vi "dms-main-train-1.vi"() -> ()   [LabVIEW 2015]
uses:
  states-enum.ctl
  <vilib>/platform/TimedLoop/XDataNode/XDataNode.xnode
  <vilib>/Platform/TimedLoop/XDataNode/nitl_modes.ctl
  <vilib>/Platform/TimedLoop/XDataNode/XDNodeRunTimeDep.lvlib
  <vilib>/Platform/TimedLoop/XDataNode/wakeup.ctl
  <vilib>/Platform/TimedLoop/XDataNode/timing_clust.ctl
  Device/Methods/Speaker-Play.vi
  Rack/Methods/Rack-Refresh.vi
  Device/Methods/Lickometer-Read.vi
  Device/Methods/Valve-Init.vi
  Device/Methods/Juicer-Init.vi
  Device/Methods/Speaker-Init.vi
  Rack/Methods/Rack-Start.vi
  Rack/Methods/Rack-Config.vi
  Device/Methods/Lickometer-Init.vi
  Rack/Methods/Rack-Init.vi
  Device/Methods/Valve-Pulse.vi
  <vilib>/Utility/file.llb/Read Delimited Spreadsheet (I64).vi
  Device/Methods/Lickometer-Stop.vi
  Rack/Methods/Rack-Stop.vi
  Rack/Typedefs/OutputRequest.ctl
  Rack/Typedefs/OutputRequest refnum.ctl
  Rack/Methods/Port drivers/DigitalInput-DataCluster.ctl
  Rack/Typedefs/InputData cluster.ctl
  Device/Typedefs/Lickometer.ctl
  Device/Typedefs/Speaker.ctl
  Device/Typedefs/Juicer.ctl
  Device/Typedefs/Valve.ctl
panel:
  out "InputData 3":T1
  out "InputData 2":T1
  in  "stop":bool
  out "Acc":dbl
  out "Time":dbl format="%#.0f"
  out "Trials":string
  out "Reward Dispensed (uL)":string
  out "Licks":string
  out "CR":string
  out "Miss":string
  out "FA":string
  out "Hits":string
  out "Current State":string
  out "Time Elapsed":dbl format="%<%H:%M:%S>t"
  in  "Tab Control":enum32{"Required", "Optional", "Devices"}(tab)
  in  "Tone Pairs":u16(ring) items=["1: 3000 Hz, 12000 Hz", "2: 5800 Hz, 5000 Hz", "3: 5000 Hz, 10000 Hz", "4: 8000 Hz, 15000 Hz"]
  in  "Max Time (s)":dbl=3600.0
  in  "Number of trials":string(combo)="500"
  in  "Max number of \nconsecutive trials":string(combo)="3"
  in  "Animal Name":string="Mouse"
  in  "Reward Vol. (uL)":dbl=5.0
  in  "Sequence Directory":path=path "C:/Users/SiapasLab/Desktop/git/wheatley"
  in  "Assay Description":string="Auditory delayed match to sample"
  in  "Recording Location":string="BI Room 146"
  in  "Trial delay (ms)":dbl=1500.0
  in  "Punish Time (s)":dbl
  in  "Trial window (ms)":dbl=1000.0
  in  "ITI lower (s)":dbl=10.0
  in  "ITI upper (s)":dbl=10.0
  in  "Min Licks":i32=1 min=1
  in  "Data Saving Directory":path=path "\\\\CA1-17\\ld8007/anesthesia/data"
  in  "Lickometer":T3={"Settings"={"Min lick duration"=1, "Port name"="bnc_panel.p0.3", "Port index"=0}, "Lick"=FALSE, "Debouncing"={"Semaphore"=refnum, "Lick start"=0}, "OutputRequest event ref"=refnum, "InputData reference"=refnum, "Active hi?"=FALSE}
  out "InputData":T1
  in  "Speaker":T6={"Settings"={"Portname"="BNC_Panel.ao0", "Index"=0, "Timestamp portname"="BNC_Panel.P0.0"}, "OutputRequest event ref"=refnum, "InputData reference"=refnum}
  in  "Juicer":T7={"Mode"=enum."Juice/reward", "Settings"={"Bleed #1 port index"=1, "Bleed #1 port name"="juicer.bleed1", "Bleed #2 port name"="juicer.bleed2", "Bleed #2 port index"=2, "Flush port name"="juicer.flush", "Flush port index"=3, "Purge port name"="juicer.purge", "Purge port index"=0, "Timestamp port name"="dsub_panel.p9.7"}, "OutputRequest event ref"=refnum, "InputData reference"=refnum}
  in  "Valve":T8={"Settings"={"Timestamp port name"="BNC_panel.P0.0", "Port name"="BNC_panel.P0.1", "Port index"=4}, "OutputRequest event ref"=refnum, "InputData reference"=refnum, "Default length (ms)"=100}
  # "Auditory delayed match to sample task (DMS)"
  # "(must be on same NI card)"
  # "(must be on same NI card)"
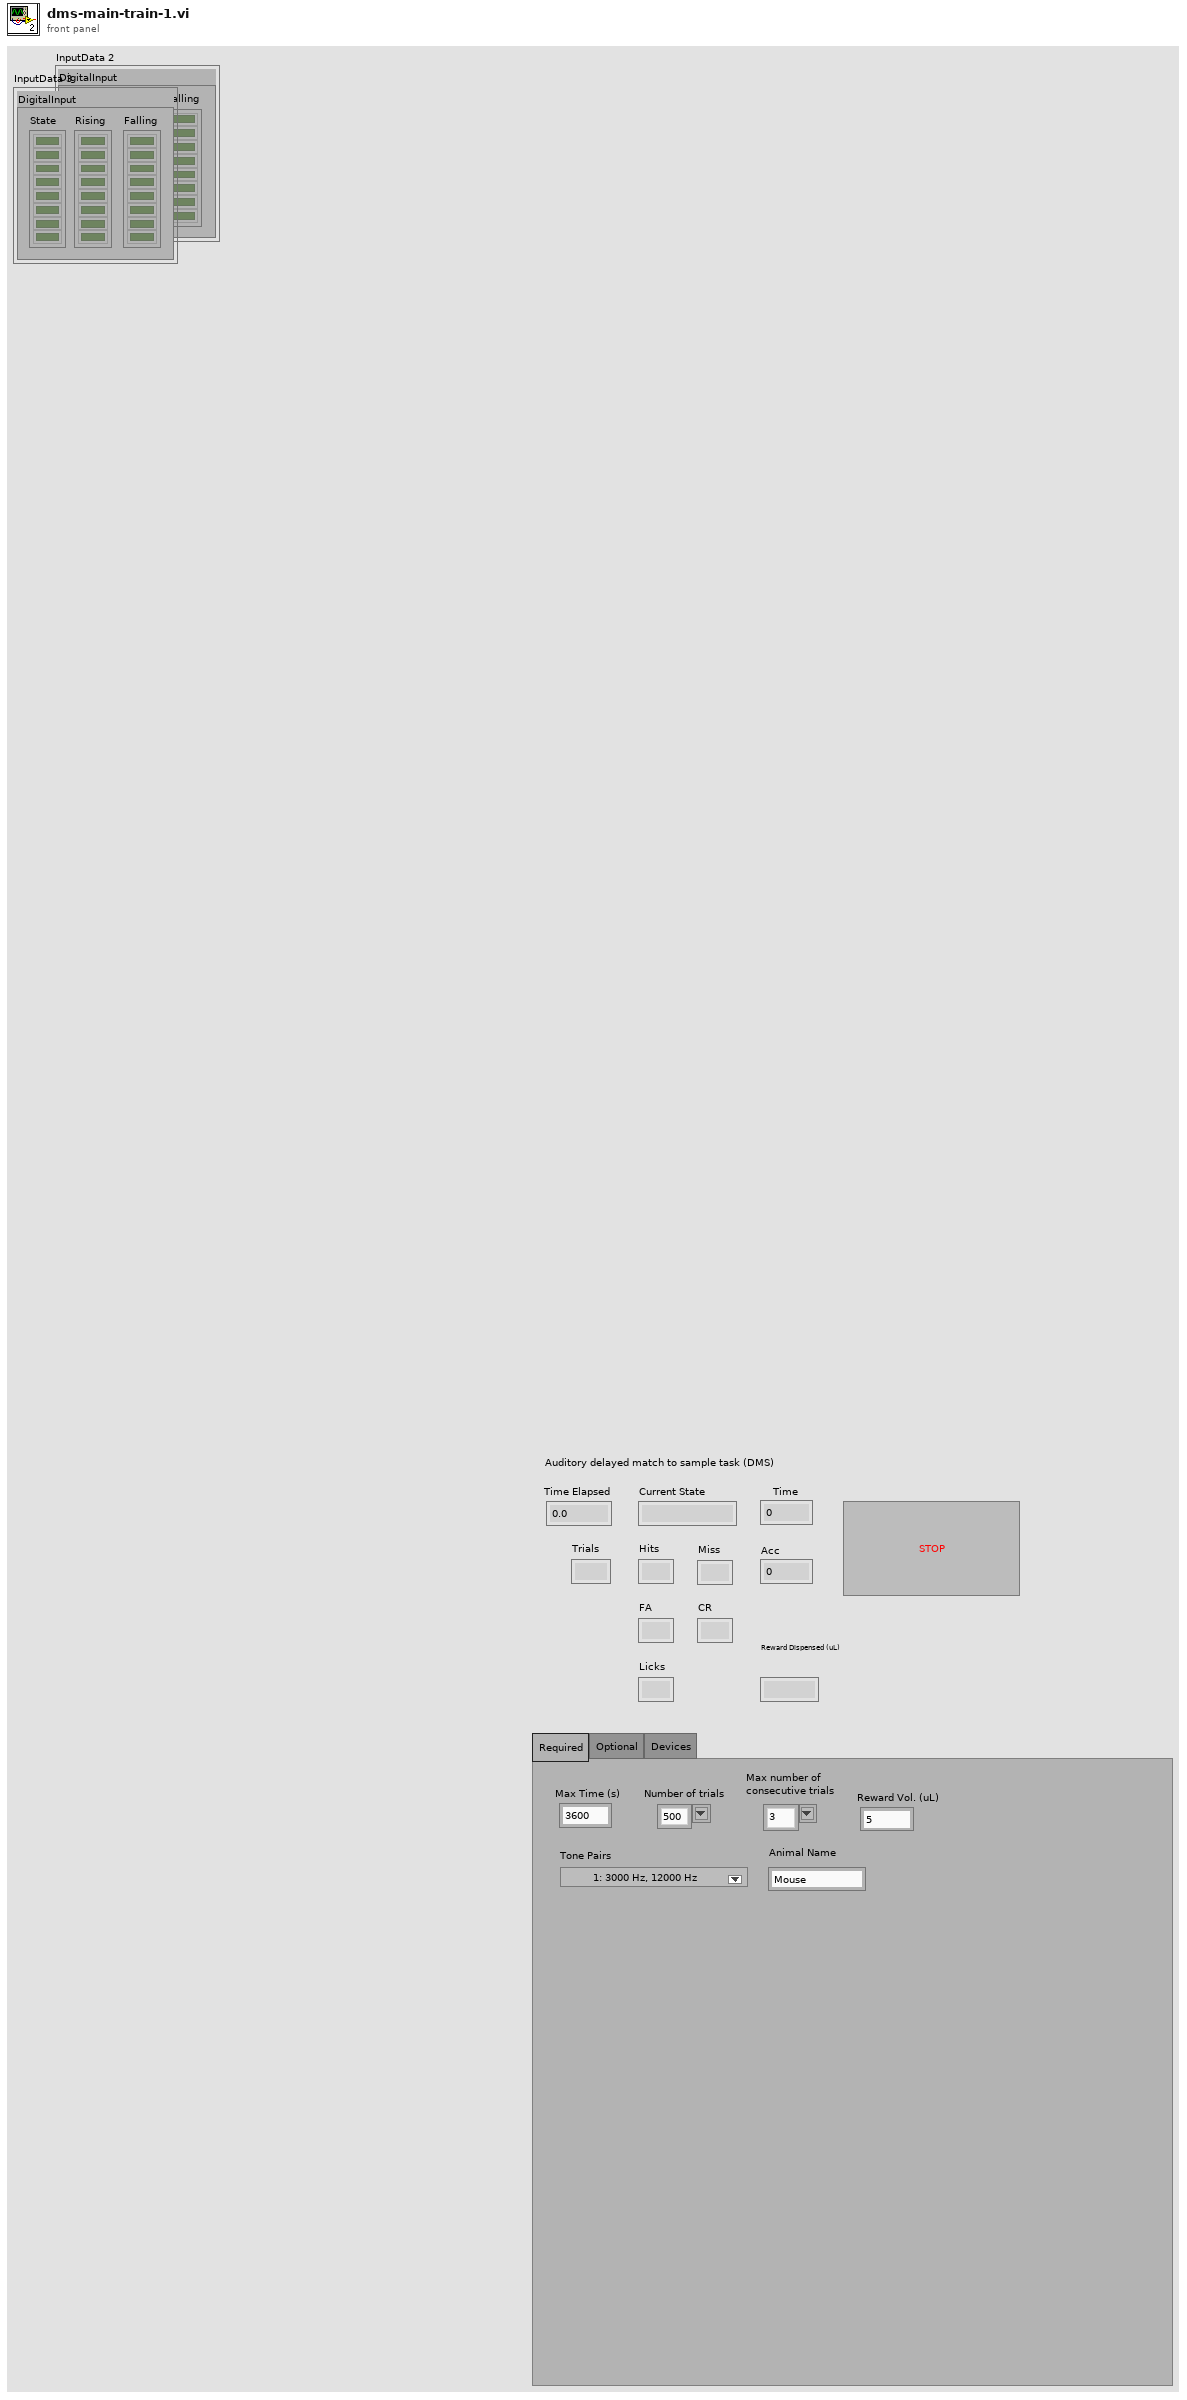
[diagram p1: front panel]
types:
  T1 = typedef "InputData cluster.ctl" = cluster{"DigitalInput":T2}
  T2 = typedef "DigitalInput-DataCluster.ctl" = cluster{"Falling":bool[], "Rising":bool[], "State":bool[]}
  T3 = typedef "Lickometer.ctl" = cluster{"Settings":cluster{"Min lick duration":u32, "Port name":string, "Port index":i32}, "Lick":bool, "Debouncing":cluster{"Semaphore":T4, "Lick start":u32}, "OutputRequest event ref":T5, "InputData reference":refnum<vi>, "Active hi?":bool}
  T4 = typedef "Semaphore RefNum" = refnum<k1>
  T5 = typedef "OutputRequest refnum.ctl" = refnum<user-event>
  T6 = typedef "Speaker.ctl" = cluster{"Settings":cluster{"Portname":string, "Index":i32, "Timestamp portname":string}, "OutputRequest event ref":T5, "InputData reference":refnum<vi>}
  T7 = typedef "Juicer.ctl" = cluster{"Mode":enum16{"Off", "Juice/reward", "Water flush", "Air purge"}, "Settings":cluster{"Bleed #1 port index":i32, "Bleed #1 port name":string, "Bleed #2 port name":string, "Bleed #2 port index":i32, "Flush port name":string, "Flush port index":i32, "Purge port name":string, "Purge port index":i32, "Timestamp port name":string}, "OutputRequest event ref":T5, "InputData reference":refnum<vi>}
  T8 = typedef "Valve.ctl" = cluster{"Settings":cluster{"Timestamp port name":string, "Port name":string, "Port index":i32}, "OutputRequest event ref":T5, "InputData reference":refnum<vi>, "Default length (ms)":i32}
  T9 = typedef "states-enum.ctl" = enum16{"ITI", "Trial", "Stop"}
  T10 = typedef "Rack driver configuration cluster.ctl" = cluster{"DigitalInput":T11, "DigitalOutput":T12, "FileOutput":T13, "AnalogOutput":T14, "DataSocketOutput":T15}
  T11 = typedef "DigitalInput-Configuration.ctl" = cluster{"Lines":tag[], "Refresh period (ms)":u32}
  T12 = typedef "DigitalOutput-Configuration.ctl" = cluster{"Output Lines":tag[], "DO timestamp lines":tag[], "Timestamp lines":tag[]}
  T13 = typedef "FileOutput-Configuration.ctl" = cluster{"Logfile path":path}
  T14 = typedef "AnalogOutput-Configuration.ctl" = cluster{"Output Lines":tag[], "AO timestamp lines":tag[]}
  T15 = typedef "DataSocketOutput-Configuration.ctl" = cluster{"DataSocket URL":string}
  T16 = cluster{"ITI upper (s)":dbl, "ITI lower (s)":dbl, "Punish Time (s)":dbl, "Trial window (ms)":dbl, "Trial delay (ms)":dbl, "Max Time (s)":dbl, "Min Licks":i32, "Reward Vol. (uL)":dbl, "Tone 1":i32, "Tone 2":i32}
  T17 = cluster{"appended path":path, "relative seconds":dbl, "Current Trial Index":i32, "Accuracy":dbl, "Hits":i32, "Miss":i32, "False Alarm":i32, "Correct Rejection":i32, "Licks":i32, "Reward Dispensed":dbl, "Punish ITI":bool, "Next Trial":i32}
  T18 = typedef "XDNodeRunTimeDep.lvlib/timing_clust.ctl" = cluster{"Expected End [f-1]":u64, "Actual End [f-1]":u64, "Finished Late? [f-1]":bool, "Expected End [i-1]":u64, "Actual End [i-1]":u64, "Finished Late? [i-1]":bool, "Expected Start [i]":u64, "Actual Start [i]":u64, "Expected Start [f]":u64, "Actual Start [f]":u64, "Source Name":string, "Structure Name":string, "Period":i64, "Deadline":i64, "Offset":i64, "Start":i64, "Priority":i32, "Timeout":i32, "Mode":T19, "Wakeup Reason":T20, "Error":errorcluster, "Source Type":string, "Secondary Source Type":string, "Global End Time":u64, "Global Start Time":u64, "Frame Duration":u64, "Iteration Duration":u64, "Assigned CPU":i32, "I/O Scan Engine Mode":u32}
  T19 = typedef "XDNodeRunTimeDep.lvlib/nitl_modes.ctl" = enum32{"No Change", "Process missed periods, maintain original phase", "Discard missed periods, maintain original phase", "Process missed periods, ignore original phase", "Discard missed periods, ignore original phase"}
  T20 = typedef "XDNodeRunTimeDep.lvlib/wakeup.ctl" = enum32{"Normal", "Aborted", "Asynchronous wakeup", "Timing source error", "Timed loop error", "Timeout"}
  T21 = cluster{"Trial Hit":bool, "Trial Miss":bool, "Trial FA":bool, "Trial CR":bool, "Skip Receiving":bool}
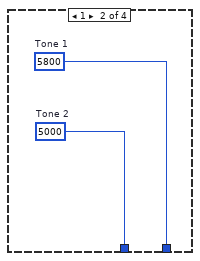
[diagram p2: hidden frame]
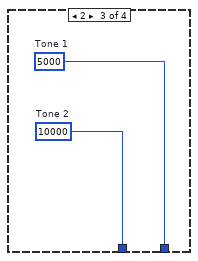
[diagram p3: hidden frame]
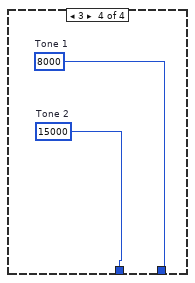
[diagram p4: hidden frame]
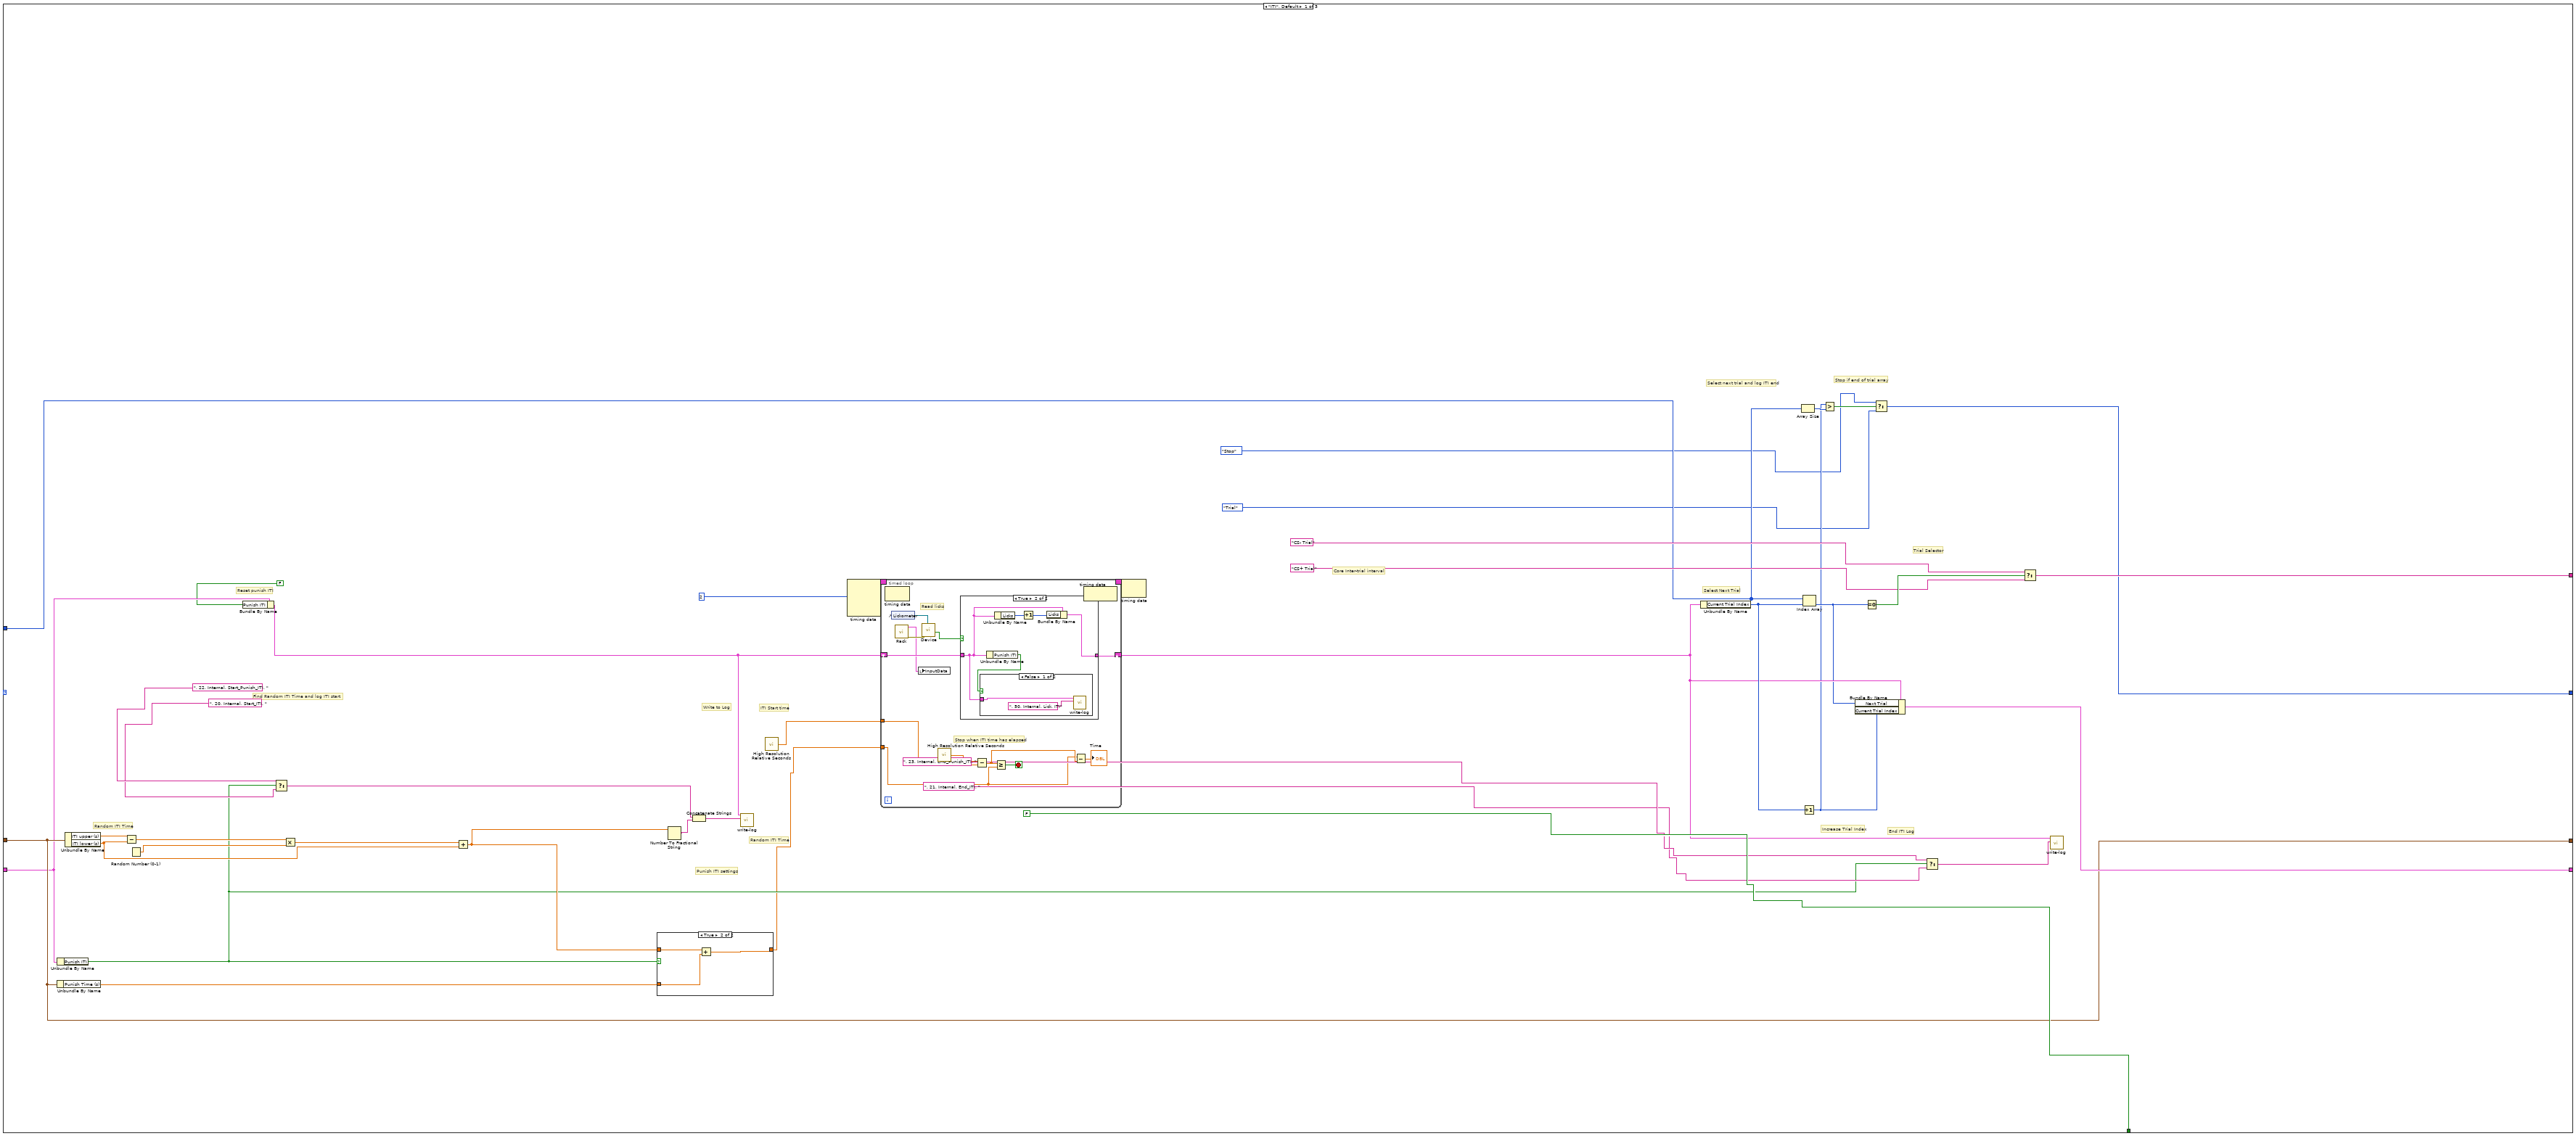
[diagram p6: hidden frame]
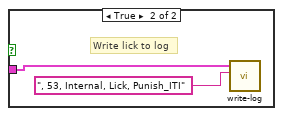
[diagram p8: hidden frame]
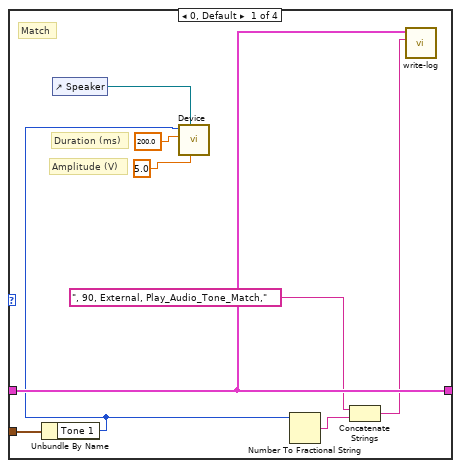
[diagram p11: hidden frame]
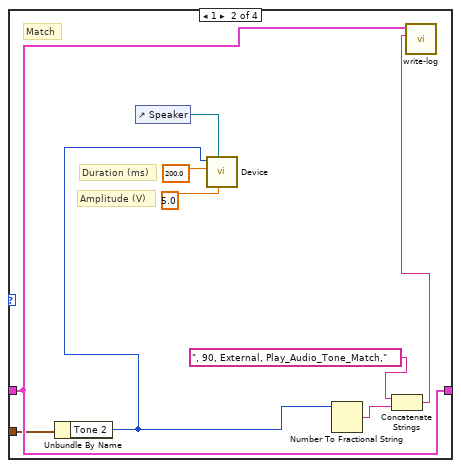
[diagram p12: hidden frame]
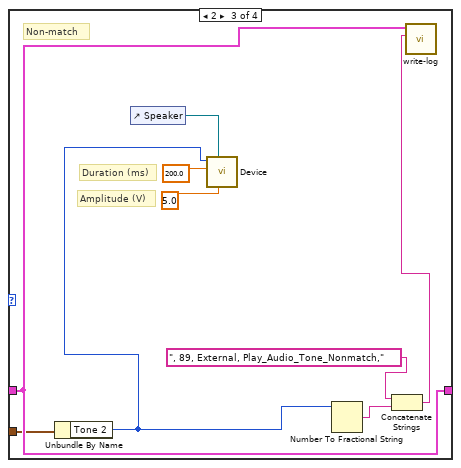
[diagram p13: hidden frame]
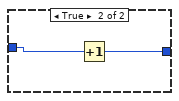
[diagram p14: hidden frame]
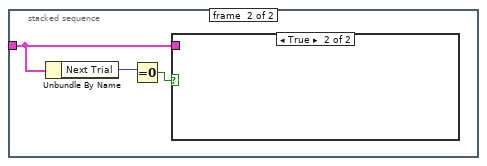
[diagram p16: hidden frame]
diagram:
  w141 = 0  # Next Trial
  w142 = FALSE  # Punish ITI
  w151 = 0.0  # Reward Dispensed
  w152 = 0  # Licks
  w153 = 0  # Correct Rejection
  w154 = 0  # False Alarm
  w157 = 0.0  # Accuracy
  w155 = 0  # Miss
  w156 = 0  # Hits
  w158 = 0  # Current Trial Index
  # "TRAINING"
  # "Create directory"
  # "Lickometer"
  # "Lickometer"
  # "Devices"
  # "Tone Pair Interpretation"
  # "Exit Logging"
  # "Front Panel Logging"
  # "CS+\nDelay lick: Miss\nReception lick: Hit\nNo lick: Miss\n\nCS-\nDelay lick: False alarm\nReception lick: False alarm\nNo lick: Correct reject"
  # "Start time"
  # "Internal Variables"
  # "External variables from Front Panel"
  # "External variable cluster"
  # "Internal variable cluster"
  # "State enum"
  # "Trial shift register"
  # "State machine"
  # "Front Panel Elements"
  # "Write trial sequence to log"
  # "Human readable time"
  # "End of header delimiter"
  # "Start Time"
  # "Environment"
  # "Schedule"
  # "Initialize data logger"
  # "Random sequence selection"
  # "Read in entire .csv"
  # "Load pre-generated sequences"
  n1 = Format Date/Time String(time format string (%c)="%Y-%m-%d-%H-%M-%S") -> (date/time string=w4:string)  [unwired: 2 in]
  n2 = case shown="0, Default" "Tone Pairs" {
    tunnel: [w224 w225 w227 w229] -> w39
    tunnel: [w223 w226 w228 w230] -> w40
    frame 0, Default {
      w224 = 12000  # Tone 2
      w223 = 3000  # Tone 1
    }
    frame 1 {
      w225 = 5000  # Tone 2
      w226 = 5800  # Tone 1
    }
    frame 2 {
      w227 = 10000  # Tone 2
      w228 = 5000  # Tone 1
    }
    frame 3 {
      w229 = 15000  # Tone 2
      w230 = 8000  # Tone 1
    }
  }
  n3 = Build Path(base path="Data Saving Directory", name or relative path=w4) -> (appended path=w2:path)
  n4 = Create Folder(path (use dialog)=w2) -> (created path=w1:path)  [unwired: 2 in, 2 out]
  n5 = control-ref of="InputData"() -> (w13:refnum<vi>)
  n6 = Build Path(base path=w1, name or relative path="data.txt") -> (appended path=w148:path)
  n7 = call-poly "Rack.vi"() -> ("error out"=w7:errorcluster, "OutputRequest\nevent ref"=w8:T5)  [unwired: 10 in]
  n8 = control-ref of="Juicer"() -> (w6:refnum<vi>)
  n9 = Path To String(path="Sequence Directory") -> (string=w96:string)
  n10 = call-poly "Device.vi"("Device reference"=w6, "error in (no error)"=w7, "OutputRequest event ref"=w8, "InputData reference"=w13) -> ("error out"=w10:errorcluster, "OutputRequest (dup)"=w15:T5, "InputData (dup)"=w12:refnum<vi>)  [unwired: 5 in]
  n11 = control-ref of="Valve"() -> (w5:refnum<vi>)
  n12 = Concatenate Strings(w96, "\\sequences\\seq_n_", "Number of trials", "_k_" ("string"), "Max number of \nconsecutive trials", "_m_2.csv" ("string")) -> (w214:string)
  n13 = call-poly "Device.vi"("Device reference"=w5, "error in (no error)"=w10, "OutputRequest event ref"=w15, "InputData reference"=w12) -> ("error out"=w9:errorcluster, "OutputRequest (dup)"=w14:T5, "InputData (dup)"=w11:refnum<vi>)  [unwired: 5 in]
  n14 = String To Path(string=w214) -> (path=w215:path)
  n15 = control-ref of="Speaker"() -> (w16:refnum<vi>)
  n16 = Concatenate Strings("Schedule," ("string"), "Assay Description", "\r\n") -> (w205:string)
  n17 = call-poly "Device.vi"("Device reference"=w16, "error in (no error)"=w9, "OutputRequest event ref"=w14, "InputData reference"=w11) -> ("error out"=w18:errorcluster, "OutputRequest (dup)"=w19:T5, "InputData (dup)"=w17:refnum<vi>)  [unwired: 5 in]
  n18 = Concatenate Strings("Path," ("string"), w96, "\r\n") -> (w99:string)
  n19 = call-poly <vilib>:"Read Delimited Spreadsheet.vi"("file path (dialog if empty)"=w215, "number of rows (all:-1)"=-1, "delimiter (\\t)"="," ("delimiter (\\t)")) -> ("all rows"=w209:i64[][])  [unwired: 7 in, 5 out]
  n20 = Write to Text File(file (use dialog)=w148, text=w205) -> (refnum out=w207:refnum<file>)  [unwired: 2 in, 2 out]
  n21 = control-ref of="Lickometer"() -> (w23:refnum<vi>)
  n22 = call-poly "Device.vi"("Device reference"=w23, "error in (no error)"=w18, "OutputRequest event ref"=w19, "InputData reference"=w17) -> ("error out"=w28:errorcluster, "OutputRequest (dup)"=w25:T5)  [unwired: 5 in, 1 out]
  n23 = Concatenate Strings("Environment," ("string"), "Recording Location", "\r\n") -> (w201:string)
  n24 = Array Size(array=w209) -> (size(s)=w213:i32[])
  n25 = Write to Text File(file (use dialog)=w207, text=w201) -> (refnum out=w101:refnum<file>)  [unwired: 2 in, 2 out]
  n26 = Format Date/Time String() -> (date/time string=w175:string)  [unwired: 3 in]
  n27 = call-poly "Rack.vi"("error in (no error)"=w28) -> ("error out"=w27:errorcluster, "Configuration"=w26:T10)  [unwired: 9 in]
  n28 = Index Array(array=w213, index=0) -> (element=w211:i32)
  n29 = Random Number (0-1)() -> (number: 0 to 1=w220:dbl)
  n30 = Write to Text File(file (use dialog)=w101, text=w99) -> (refnum out=w100:refnum<file>)  [unwired: 2 in, 2 out]
  n31 = Decrement(x=w211) -> (x-1=w210:i32)
  n32 = call-poly "Rack.vi"("error in (no error)"=w27, "OutputRequest event ref"=w25, "Configuration"=w26) -> ("OutputRequest event ref (dup)"=w21:T5)  [unwired: 7 in, 1 out]
  n33 = Multiply(x=w220, y=w210) -> (x*y=w219:dbl)
  n34 = Concatenate Strings("Time," ("string"), w175, "\r\n") -> (w197:string)
  n35 = To Long Integer(number=w219) -> (32bit integer=w208:i32)
  n36 = Write to Text File(file (use dialog)=w100, text=w197) -> (refnum out=w196:refnum<file>)  [unwired: 2 in, 2 out]
  n37 = call <vilib>:"High Resolution Relative Seconds.vi"() -> ("relative seconds"=w160:dbl)
  n38 = Index Array(array=w209, index (row)=w208) -> (element=w150:i64[])  [unwired: 1 in]
  n39 = Bundle("ITI upper (s)"="ITI upper (s)", "ITI lower (s)"="ITI lower (s)", "Punish Time (s)"="Punish Time (s)", "Trial window (ms)"="Trial window (ms)", "Trial delay (ms)"="Trial delay (ms)", "Max Time (s)"="Max Time (s)", "Min Licks"="Min Licks", "Reward Vol. (uL)"="Reward Vol. (uL)", "Tone 1"=w40, "Tone 2"=w39) -> (w135:T16)  [unwired: 1 in]
  n40 = Concatenate Strings("Animal," ("string"), "Animal Name", "\r\n") -> (w193:string)
  n41 = Unbundle By Name(w135) -> ("Max Time (s)"=w134:dbl, "Trial delay (ms)"=w133:dbl, "Trial window (ms)"=w132:dbl, "ITI lower (s)"=w131:dbl, "ITI upper (s)"=w130:dbl, "Punish Time (s)"=w129:dbl, "Min Licks"=w52:i32, "Reward Vol. (uL)"=w44:dbl, "Tone 1"=w32:i32, "Tone 2"=w31:i32)
  n42 = Write to Text File(file (use dialog)=w196, text=w193) -> (refnum out=w185:refnum<file>)  [unwired: 2 in, 2 out]
  n43 = Bundle("appended path"=w148, "relative seconds"=w160, "Current Trial Index"=w158, "Accuracy"=w157, "Hits"=w156, "Miss"=w155, "False Alarm"=w154, "Correct Rejection"=w153, "Licks"=w152, "Reward Dispensed"=w151, "Punish ITI"=w142, "Next Trial"=w141) -> (w159:T17)  [unwired: 1 in]
  n44 = for {
    N -> [w232]
    shift-right: [w236] -> w140
    shift-left: " " -> [w237]
    tunnel: w150 -> [w239] mode=indexing
    i -> [w235]
    n45 = Decrement(x=w232) -> (x-1=w231:i32)
    n46 = Equal?(x=w231, y=w235) -> (x = y?=w234:bool)
    n47 = Number To Decimal String(number=w239) -> (decimal integer string=w238:string)  [unwired: 1 in]
    n48 = case shown="False" w234 {
      tunnel: [", " ("string") "" ("string")] -> w233
      frame False {
      }
      frame True {
      }
    }
    n49 = Concatenate Strings(w237, w238, w233) -> (w236:string)
  }
  n50 = Concatenate Strings("Trials," ("string"), "Number of trials", "\r\n") -> (w189:string)
  n51 = Write to Text File(file (use dialog)=w185, text=w189) -> (refnum out=w184:refnum<file>)  [unwired: 2 in, 2 out]
  n52 = Number To Fractional String(number=w32) -> (F-format string=w33:string)  [unwired: 3 in]
  n53 = Number To Fractional String(number=w44) -> (F-format string=w43:string)  [unwired: 3 in]
  n54 = Number To Fractional String(number=w31) -> (F-format string=w34:string)  [unwired: 3 in]
  n55 = Number To Fractional String(number=w134) -> (F-format string=w128:string)  [unwired: 3 in]
  n56 = Number To Fractional String(number=w129) -> (F-format string=w116:string)  [unwired: 3 in]
  n57 = Number To Fractional String(number=w52) -> (F-format string=w51:string)  [unwired: 3 in]
  n58 = Number To Fractional String(number=w133) -> (F-format string=w125:string)  [unwired: 3 in]
  n59 = Number To Fractional String(number=w132) -> (F-format string=w122:string)  [unwired: 3 in]
  n60 = Number To Fractional String(number=w131) -> (F-format string=w121:string)  [unwired: 3 in]
  n61 = Number To Fractional String(number=w130) -> (F-format string=w119:string)  [unwired: 3 in]
  n62 = Concatenate Strings("Max_Time_s," ("string"), w128, "\r\n") -> (w110:string)
  n63 = Concatenate Strings("Consecutive_Trials," ("string"), "Max number of \nconsecutive trials", "\r\n") -> (w186:string)
  n64 = Concatenate Strings("CS+_Tone," ("string"), w33, "\r\n") -> (w30:string)
  n65 = Concatenate Strings("Min_Licks," ("string"), w51, "\r\n") -> (w48:string)
  n66 = Concatenate Strings("Reward_Volume," ("string"), w43, "\r\n") -> (w42:string)
  n67 = Concatenate Strings("CS-_Tone," ("string"), w34, "\r\n") -> (w29:string)
  n68 = Concatenate Strings("Delay_Window_ms," ("string"), w125, "\r\n") -> (w109:string)
  n69 = Concatenate Strings("ITI_Lower_s," ("string"), w121, "\r\n") -> (w107:string)
  n70 = Concatenate Strings("Reception_Window_ms," ("string"), w122, "\r\n") -> (w108:string)
  n71 = Concatenate Strings("ITI_Upper_s," ("string"), w119, "\r\n") -> (w106:string)
  n72 = Concatenate Strings("Punish_Time_s," ("string"), w116, "\r\n") -> (w105:string)
  n73 = Write to Text File(file (use dialog)=w184, text=w186) -> (refnum out=w104:refnum<file>)  [unwired: 2 in, 2 out]
  n74 = while {
    shift-right: [w275] -> _
    shift-left: states-enum."ITI" -> [w252]
    shift-right: [w251] -> _
    shift-left: w135 -> [w267]
    shift-right: [w266] -> w60
    shift-left: w159 -> [w246]
    tunnel: w150 -> [w269]
    tunnel: w21 -> [w245]
    tunnel: [w245] -> w20
    stop <- w247 stop-if-true
    # "State enum"
    # "Internal variable cluster"
    # "External variable cluster"
    # "Update front panel"
    # "Update front panel"
    # "Wait for current state to finish before ending session"
    n75 = case shown="\"Trial\"" w252 {
      tunnel: [w294 states-enum."ITI" states-enum."Stop"] -> w275
      tunnel: [FALSE FALSE TRUE] -> w271
      tunnel: w269 -> [w299 _ _]
      tunnel: [w303 w403 "Stop"] -> w268
      tunnel: w267 -> [w302 w356 w750]
      tunnel: [w308 w369 w746] -> w266
      tunnel: w246 -> [w293 w372 w746]
      tunnel: [w302 w356 w750] -> w251
      frame "ITI", Default {
        # "Reset punish ITI"
        # "Stop if end of trial array"
        # "Punish ITI settings"
        # "Select next trial and log ITI end"
        # "Trial Selector"
        # "Increase Trial Index"
        # "Select Next Trial"
        # "End ITI Log"
        # "ITI Start time"
        # "Core Inter-trial interval"
        # "Find Random ITI Time and log ITI start"
        # "Random ITI Time"
        # "Write to Log"
        # "Random ITI Time"
        n76 = Unbundle By Name(w302) -> ("Punish Time (s)"=w301:dbl)
        n77 = Unbundle By Name(w293) -> ("Punish ITI"=w284:bool)
        n78 = Unbundle By Name(w302) -> ("ITI upper (s)"=w311:dbl, "ITI lower (s)"=w315:dbl)
        n79 = Subtract(x=w311, y=w315) -> (x-y=w312:dbl)
        n80 = Random Number (0-1)() -> (number: 0 to 1=w313:dbl)
        n81 = Bundle By Name(cluster=w293, "Punish ITI"=FALSE) -> (w292:T17)
        n82 = Select(t=", 22, Internal, Start_Punish_ITI, " ("text"), s=w284, f=", 20, Internal, Start_ITI, " ("text")) -> (s? t:f=w288:string)
        n83 = Multiply(x=w312, y=w313) -> (x*y=w314:dbl)
        n84 = Add(x=w314, y=w315) -> (x+y=w300:dbl)
        n85 = case shown="True" w284 {
          tunnel: w300 -> [w347 w350]
          tunnel: [w347 w349] -> w282
          tunnel: w301 -> [_ w348]
          frame False {
          }
          frame True {
            n86 = Add(x=w350, y=w348) -> (x+y=w349:dbl)
          }
        }
        n87 = Number To Fractional String(number=w300) -> (F-format string=w317:string)  [unwired: 3 in]
        n88 = Concatenate Strings(w288, w317) -> (w316:string)
        n89 = call "write-log.vi"("Write Text"=w316, "Internal Cluster"=w292) -> ()  [unwired: 10 in]
        n90 = call <vilib>:"High Resolution Relative Seconds.vi"() -> ("relative seconds"=w283:dbl)
        n91 = node-c288(i64 2 ("Period")) -> (w281:T18)  [unwired: 3 in]
        n92 = timed-loop {
          tunnel: w282 -> [w323]
          tunnel: w283 -> [w324]
          shift-right: [w327] -> w309
          shift-left: w292 -> [w328]
          timing: w281 -> [_]
          timing-out: [_] -> w280
          stop <- w329 stop-if-true
          # "Read licks"
          # "Stop when ITI time has elapsed"
          n93 = node-c288() -> ()  [unwired: 1 in, 1 out]
          n94 = control-ref of="Lickometer"() -> (w322:refnum<vi>)
          n95 = call-poly "Rack.vi"() -> ("error out"=w321:errorcluster, "Data Cluster"=w319:T1)  [unwired: 10 in]
          n96 = local write "InputData"(w319) -> ()
          n97 = call-poly "Device.vi"("Device reference"=w322, "error in (no error)"=w321) -> ("Lick start?"=w320:bool)  [unwired: 7 in, 2 out]
          n98 = call <vilib>:"High Resolution Relative Seconds.vi"() -> ("relative seconds"=w330:dbl)
          n99 = case shown="True" w320 {
            tunnel: w328 -> [w333 w334]
            tunnel: [w333 w336] -> w327
            frame False {
            }
            frame True {
              n100 = Unbundle By Name(w334) -> ("Punish ITI"=w335:bool)
              n101 = case shown="False" w335 {
                tunnel: w334 -> [w340 w341]
                frame False {
                  n102 = call "write-log.vi"("Write Text"=", 50, Internal, Lick, ITI" ("text"), "Internal Cluster"=w340) -> ()  [unwired: 10 in]
                }
                frame True {
                  # "Write lick to log"
                  n103 = call "write-log.vi"("Write Text"=", 53, Internal, Lick, Punish_ITI" ("text"), "Internal Cluster"=w341) -> ()  [unwired: 10 in]
                }
              }
              n104 = Unbundle By Name(w334) -> ("Licks"=w338:i32)
              n105 = Increment(x=w338) -> (x+1=w337:i32)
              n106 = Bundle By Name(cluster=w334, "Licks"=w337) -> (w336:T17)
            }
          }
          n107 = Subtract(x=w330, y=w324) -> (x-y=w325:dbl)
          n108 = Greater Or Equal?(x=w325, y=w323) -> (x >= y?=w329:bool)
          n109 = Subtract(x=w323, y=w325) -> (x-y=→"Time":dbl)
          n110 = node-c288() -> ()  [unwired: 1 in, 1 out]
        }
        n111 = node-c288(w280) -> ()  [unwired: 1 out]
        n112 = Unbundle By Name(w309) -> ("Current Trial Index"=w310:i32)
        n113 = Array Size(array=w299) -> (size(s)=w298:i32)
        n114 = Increment(x=w310) -> (x+1=w297:i32)
        n115 = Index Array(array=w299, index=w310) -> (element=w307:i64)
        n116 = Greater?(x=w297, y=w298) -> (0:w296:bool)
        n117 = Bundle By Name(cluster=w309, "Next Trial"=w307, "Current Trial Index"=w297) -> (w308:T17)
        n118 = Equal To 0?(x=w307) -> (x = 0?=w306:bool)
        n119 = Select(t=states-enum."Stop", s=w296, f=states-enum."Trial") -> (s? t:f=w294:T9)
        n120 = Select(t=", 23, Internal, End_Punish_ITI, " ("text"), s=w284, f=", 21, Internal, End_ITI, " ("text")) -> (s? t:f=w287:string)
        n121 = Select(t="CS- Trial", s=w306, f="CS+ Trial") -> (s? t:f=w303:string)
        n122 = call "write-log.vi"("Write Text"=w287, "Internal Cluster"=w309) -> ()  [unwired: 10 in]
      }
      frame "Trial" {
        w374 = 0  # Current Number Reception Licks
        w375 = 0  # Current Number Delay Licks
        w377 = FALSE  # Skip Receiving
        # "TRAINING"
        # "Only reward hit"
        # "Log metrics"
        # "Trial Window Log"
        # "Dispense reward"
        # "Enable punishment if FA or CR"
        # "Accuracy"
        # "Update metrics using local cluster"
        # "S+ No Lick - Miss\nS- No Lick - Correct Reject"
        # "Convert to s"
        # "Trial Reception Window"
        # "Convert to s"
        # "Trial Start Time"
        # "Trial Delay"
        n123 = node-c288(i64 2 ("Period")) -> (w367:T18)  [unwired: 3 in]
        n124 = Unbundle By Name(w372) -> ("Next Trial"=w352:i32)
        n125 = case shown="3" w352 {
          tunnel: w372 -> [w710 w712 w714 w716]
          tunnel: [w710 w712 w714 w716] -> w371
          frame 0, Default {
            # "Match"
            n126 = call "write-log.vi"("Write Text"=", 95, Internal, Start_Match_Trial, " ("text"), "Internal Cluster"=w710) -> ()  [unwired: 10 in]
          }
          frame 1 {
            # "Match"
            n127 = call "write-log.vi"("Write Text"=", 95, Internal, Start_Match_Trial, " ("text"), "Internal Cluster"=w712) -> ()  [unwired: 10 in]
          }
          frame 2 {
            # "Non-match"
            n128 = call "write-log.vi"("Write Text"=", 96, Internal, Start_Nonmatch_Trial, " ("text"), "Internal Cluster"=w714) -> ()  [unwired: 10 in]
          }
          frame 3 {
            # "Nonmatch"
            n129 = call "write-log.vi"("Write Text"=", 96, Internal, Start_Nonmatch_Trial, " ("text"), "Internal Cluster"=w716) -> ()  [unwired: 10 in]
          }
        }
        n130 = timed-loop {
          tunnel: w371 -> [w647]
          tunnel: [w641] -> w431
          tunnel: w356 -> [w646]
          timing: w367 -> [_]
          timing-out: [_] -> w366
          stop <- TRUE stop-if-true
          # "Read Speaker Lick"
          # "Play Sound While Loop"
          n131 = node-c288() -> ()  [unwired: 1 in, 1 out]
          n132 = Unbundle By Name(w647) -> ("Next Trial"=w639:i32)
          n133 = case shown="1" w639 {
            tunnel: w647 -> [w665 w674 w683 w692]
            tunnel: [w665 w674 w683 w692] -> w642
            tunnel: w646 -> [w664 w670 w679 w688]
            frame 0, Default {
              # "Duration (ms)"
              # "Amplitude (V)"
              # "Match"
              n134 = Unbundle By Name(w664) -> ("Tone 1"=w657:i32)
              n135 = control-ref of="Speaker"() -> (w658:refnum<vi>)
              n136 = call-poly "Device.vi"("Amplitude (V)"=5.0, "Device reference"=w658, "Duration (ms)"=200.0, "Frequency (Hz)"=w657) -> ()  [unwired: 7 in, 1 out]
              n137 = Number To Fractional String(number=w657) -> (F-format string=w663:string)  [unwired: 3 in]
              n138 = Concatenate Strings(", 90, External, Play_Audio_Tone_Match," ("text"), w663) -> (w661:string)
              n139 = call "write-log.vi"("Write Text"=w661, "Internal Cluster"=w665) -> ()  [unwired: 10 in]
            }
            frame 1 {
              # "Duration (ms)"
              # "Amplitude (V)"
              # "Match"
              n140 = Unbundle By Name(w670) -> ("Tone 2"=w666:i32)
              n141 = control-ref of="Speaker"() -> (w667:refnum<vi>)
              n142 = call-poly "Device.vi"("Amplitude (V)"=5.0, "Device reference"=w667, "Duration (ms)"=200.0, "Frequency (Hz)"=w666) -> ()  [unwired: 7 in, 1 out]
              n143 = Number To Fractional String(number=w666) -> (F-format string=w671:string)  [unwired: 3 in]
              n144 = Concatenate Strings(", 90, External, Play_Audio_Tone_Match," ("text"), w671) -> (w672:string)
              n145 = call "write-log.vi"("Write Text"=w672, "Internal Cluster"=w674) -> ()  [unwired: 10 in]
            }
            frame 2 {
              # "Duration (ms)"
              # "Amplitude (V)"
              # "Non-match"
              n146 = Unbundle By Name(w679) -> ("Tone 1"=w675:i32)
              n147 = control-ref of="Speaker"() -> (w676:refnum<vi>)
              n148 = call-poly "Device.vi"("Amplitude (V)"=5.0, "Device reference"=w676, "Duration (ms)"=200.0, "Frequency (Hz)"=w675) -> ()  [unwired: 7 in, 1 out]
              n149 = Number To Fractional String(number=w675) -> (F-format string=w680:string)  [unwired: 3 in]
              n150 = Concatenate Strings(", 89, External, Play_Audio_Tone_Nonmatch," ("text"), w680) -> (w681:string)
              n151 = call "write-log.vi"("Write Text"=w681, "Internal Cluster"=w683) -> ()  [unwired: 10 in]
            }
            frame 3 {
              # "Duration (ms)"
              # "Amplitude (V)"
              # "Non-match"
              n152 = Unbundle By Name(w688) -> ("Tone 2"=w684:i32)
              n153 = control-ref of="Speaker"() -> (w685:refnum<vi>)
              n154 = call-poly "Device.vi"("Amplitude (V)"=5.0, "Device reference"=w685, "Duration (ms)"=200.0, "Frequency (Hz)"=w684) -> ()  [unwired: 7 in, 1 out]
              n155 = Number To Fractional String(number=w684) -> (F-format string=w689:string)  [unwired: 3 in]
              n156 = Concatenate Strings(", 89, External, Play_Audio_Tone_Nonmatch," ("text"), w689) -> (w690:string)
              n157 = call "write-log.vi"("Write Text"=w690, "Internal Cluster"=w692) -> ()  [unwired: 10 in]
            }
          }
          n158 = call-poly "Rack.vi"() -> ("error out"=w645:errorcluster, "Data Cluster"=w643:T1)  [unwired: 10 in]
          n159 = local write "InputData"(w643) -> ()
          n160 = control-ref of="Lickometer"() -> (w644:refnum<vi>)
          n161 = call-poly "Device.vi"("Device reference"=w644, "error in (no error)"=w645) -> ("Lick start?"=w640:bool)  [unwired: 7 in, 2 out]
          n162 = case shown="True" w640 {
            tunnel: w642 -> [w649 w650]
            tunnel: [w649 w654] -> w641
            frame False {
            }
            frame True {
              n163 = Unbundle By Name(w650) -> ("Licks"=w653:i32)
              n164 = Increment(x=w653) -> (x+1=w652:i32)
              n165 = Bundle By Name(cluster=w650, "Licks"=w652) -> (w654:T17)
              n166 = call "write-log.vi"("Write Text"=", 53, Internal, Lick, Speaker-1" ("text"), "Internal Cluster"=w650) -> ()  [unwired: 10 in]
            }
          }
          n167 = node-c288() -> ()  [unwired: 1 in, 1 out]
        }
        n168 = Unbundle By Name(w356) -> ("Min Licks"=w373:i32, "Trial delay (ms)"=w405:dbl, "Trial window (ms)"=w397:dbl)
        n169 = call <vilib>:"High Resolution Relative Seconds.vi"() -> ("relative seconds"=w406:dbl)
        n170 = case shown="3" w352 {
          tunnel: [w732 w736 w740 w744] -> w430
          tunnel: [w731 w735 w739 w743] -> w429
          tunnel: [w730 w734 w738 w742] -> w428
          tunnel: [w729 w733 w737 w741] -> w427
          frame 0, Default {
            w729 = FALSE  # Trial CR
            w730 = FALSE  # Trial FA
            w731 = TRUE  # Trial Miss
            w732 = FALSE  # Trial Hit
            # "Match"
          }
          frame 1 {
            w733 = FALSE  # Trial CR
            w734 = FALSE  # Trial FA
            w735 = TRUE  # Trial Miss
            w736 = FALSE  # Trial Hit
            # "Match"
          }
          frame 2 {
            w737 = TRUE  # Trial CR
            w738 = FALSE  # Trial FA
            w739 = FALSE  # Trial Miss
            w740 = FALSE  # Trial Hit
            # "Nonmatch"
          }
          frame 3 {
            w741 = TRUE  # Trial CR
            w742 = FALSE  # Trial FA
            w743 = FALSE  # Trial Miss
            w744 = FALSE  # Trial Hit
            # "Nonmatch"
          }
        }
        n171 = Add(x=w405, y=w397) -> (x+y=w404:dbl)
        n172 = Bundle("Trial Hit"=w430, "Trial Miss"=w429, "Trial FA"=w428, "Trial CR"=w427, "Skip Receiving"=w377) -> (w426:T21)  [unwired: 1 in]
        n173 = Divide(x=w405, y=1000.0) -> (x/y=w434:dbl)
        n174 = node-c288(w366) -> ()  [unwired: 1 out]
        n175 = node-c288(i64 2 ("Period")) -> (w364:T18)  [unwired: 3 in]
        n176 = timed-loop {
          tunnel: w434 -> [w592]
          tunnel: w406 -> [w607]
          shift-right: [w608] -> w355
          shift-left: w431 -> [w601]
          shift-right: [w605] -> w425
          shift-left: w426 -> [w606]
          tunnel: w373 -> [w597]
          shift-right: [w599] -> _
          shift-left: w375 -> [w600]
          timing: w364 -> [_]
          timing-out: [_] -> w363
          i -> [w604]
          stop <- w602 stop-if-true
          # "Min Lick Counter"
          # "Read licks"
          n177 = node-c288() -> ()  [unwired: 1 in, 1 out]
          n178 = call-poly "Rack.vi"() -> ("error out"=w595:errorcluster, "Data Cluster"=w593:T1)  [unwired: 10 in]
          n179 = control-ref of="Lickometer"() -> (w594:refnum<vi>)
          n180 = local write "InputData"(w593) -> ()
          n181 = call-poly "Device.vi"("Device reference"=w594, "error in (no error)"=w595) -> ("Lick start?"=w596:bool)  [unwired: 7 in, 2 out]
          n182 = case shown="True" w596 {
            tunnel: w600 -> [w612 w614]
            tunnel: [w612 w613] -> w599
            frame False {
            }
            frame True {
              n183 = Increment(x=w614) -> (x+1=w613:i32)
            }
          }
          n184 = Greater Or Equal?(x=w599, y=w597) -> (x >= y?=w598:bool)
          n185 = call <vilib>:"High Resolution Relative Seconds.vi"() -> ("relative seconds"=w609:dbl)
          n186 = Subtract(x=w609, y=w607) -> (x-y=w591:dbl)
          n187 = Subtract(x=w592, y=w591) -> (x-y=w590:dbl)
          n188 = local write "Time"(w590) -> ()
          n189 = case shown="True" w596 {
            tunnel: w601 -> [w628 w630]
            tunnel: [w628 w631] -> w608
            tunnel: w606 -> [w627 w629]
            tunnel: [w627 w629] -> w605
            tunnel: w598 -> [_ _]
            frame False {
            }
            frame True {
              # "Do nothing if licking during delay"
              # "If a lick is received"
              # "Write lick to log"
              n190 = Unbundle By Name(w630) -> ("Licks"=w633:i32)
              n191 = Increment(x=w633) -> (x+1=w632:i32)
              n192 = Bundle By Name(cluster=w630, "Licks"=w632) -> (w631:T17)
              n193 = call "write-log.vi"("Write Text"=", 51, Internal, Lick, Trial_Delay" ("text"), "Internal Cluster"=w630) -> ()  [unwired: 10 in]
            }
          }
          n194 = Greater Or Equal?(x=w591, y=w592) -> (x >= y?=w602:bool)
          n195 = case shown="True" w602 {
            tunnel: w601 -> [_ w616]
            frame False {
            }
            frame True {
              # "Exit Log"
              n196 = call "write-log.vi"("Write Text"=", 93, Internal, End_Trial_Delay_Window, " ("text"), "Internal Cluster"=w616) -> ()  [unwired: 10 in]
            }
          }
          n197 = Equal To 0?(x=w604) -> (x = 0?=w603:bool)
          n198 = case shown="True" w603 {
            tunnel: w601 -> [_ w617]
            tunnel: w592 -> [_ w618]
            frame False {
            }
            frame True {
              n199 = stacked-sequence {
                tunnel: w618 -> [_ w622]
                tunnel: w617 -> [w620 w623]
                frame #0 {
                  n200 = Unbundle By Name(w620) -> ("Next Trial"=w621:i32)
                  n201 = Equal To 0?(x=w621) -> (x = 0?=w619:bool)
                  n202 = case shown="False" w619 {
                    tunnel: w620 -> [_ _]
                    frame False {
                      # "CS+"
                    }
                    frame True {
                      # "CS-"
                    }
                  }
                }
                frame #1 {
                  n203 = Number To Fractional String(number=w622) -> (F-format string=w624:string)  [unwired: 3 in]
                  n204 = Concatenate Strings(", 91, Internal, Start_Trial_Delay_Window, " ("text"), w624) -> (w625:string)
                  n205 = call "write-log.vi"("Write Text"=w625, "Internal Cluster"=w623) -> ()  [unwired: 10 in]
                }
              }
            }
          }
          n206 = node-c288() -> ()  [unwired: 1 in, 1 out]
        }
        n207 = Unbundle By Name(w356) -> ("Reward Vol. (uL)"=w370:dbl)
        n208 = node-c288(w363) -> ()  [unwired: 1 out]
        n209 = node-c288() -> (w358:T18)  [unwired: 4 in]
        n210 = timed-loop {
          tunnel: w355 -> [w446]
          tunnel: [w442] -> w354
          tunnel: w356 -> [w445]
          timing: w358 -> [_]
          timing-out: [_] -> w357
          stop <- TRUE stop-if-true
          # "Read Speaker Lick"
          # "Play Sound While Loop"
          n211 = node-c288() -> ()  [unwired: 1 in, 1 out]
          n212 = Unbundle By Name(w446) -> ("Next Trial"=w440:i32)
          n213 = case shown="3" w440 {
            tunnel: w446 -> [w464 w473 w482 w491]
            tunnel: [w464 w473 w482 w491] -> w443
            tunnel: w445 -> [w463 w469 w478 w487]
            frame 0, Default {
              # "Duration (ms)"
              # "Amplitude (V)"
              # "Match"
              n214 = Unbundle By Name(w463) -> ("Tone 1"=w457:i32)
              n215 = control-ref of="Speaker"() -> (w456:refnum<vi>)
              n216 = call-poly "Device.vi"("Amplitude (V)"=5.0, "Device reference"=w456, "Duration (ms)"=200.0, "Frequency (Hz)"=w457) -> ()  [unwired: 7 in, 1 out]
              n217 = Number To Fractional String(number=w457) -> (F-format string=w462:string)  [unwired: 3 in]
              n218 = Concatenate Strings(", 90, External, Play_Audio_Tone_Match," ("text"), w462) -> (w460:string)
              n219 = call "write-log.vi"("Write Text"=w460, "Internal Cluster"=w464) -> ()  [unwired: 10 in]
            }
            frame 1 {
              # "Duration (ms)"
              # "Amplitude (V)"
              # "Match"
              n220 = Unbundle By Name(w469) -> ("Tone 2"=w466:i32)
              n221 = control-ref of="Speaker"() -> (w465:refnum<vi>)
              n222 = call-poly "Device.vi"("Amplitude (V)"=5.0, "Device reference"=w465, "Duration (ms)"=200.0, "Frequency (Hz)"=w466) -> ()  [unwired: 7 in, 1 out]
              n223 = Number To Fractional String(number=w466) -> (F-format string=w470:string)  [unwired: 3 in]
              n224 = Concatenate Strings(", 90, External, Play_Audio_Tone_Match," ("text"), w470) -> (w471:string)
              n225 = call "write-log.vi"("Write Text"=w471, "Internal Cluster"=w473) -> ()  [unwired: 10 in]
            }
            frame 2 {
              # "Duration (ms)"
              # "Amplitude (V)"
              # "Non-match"
              n226 = Unbundle By Name(w478) -> ("Tone 2"=w475:i32)
              n227 = control-ref of="Speaker"() -> (w474:refnum<vi>)
              n228 = call-poly "Device.vi"("Amplitude (V)"=5.0, "Device reference"=w474, "Duration (ms)"=200.0, "Frequency (Hz)"=w475) -> ()  [unwired: 7 in, 1 out]
              n229 = Number To Fractional String(number=w475) -> (F-format string=w479:string)  [unwired: 3 in]
              n230 = Concatenate Strings(", 89, External, Play_Audio_Tone_Nonmatch," ("text"), w479) -> (w480:string)
              n231 = call "write-log.vi"("Write Text"=w480, "Internal Cluster"=w482) -> ()  [unwired: 10 in]
            }
            frame 3 {
              # "Duration (ms)"
              # "Amplitude (V)"
              # "Non-match"
              n232 = Unbundle By Name(w487) -> ("Tone 1"=w484:i32)
              n233 = control-ref of="Speaker"() -> (w483:refnum<vi>)
              n234 = call-poly "Device.vi"("Amplitude (V)"=5.0, "Device reference"=w483, "Duration (ms)"=200.0, "Frequency (Hz)"=w484) -> ()  [unwired: 7 in, 1 out]
              n235 = Number To Fractional String(number=w484) -> (F-format string=w488:string)  [unwired: 3 in]
              n236 = Concatenate Strings(", 89, External, Play_Audio_Tone_Nonmatch," ("text"), w488) -> (w489:string)
              n237 = call "write-log.vi"("Write Text"=w489, "Internal Cluster"=w491) -> ()  [unwired: 10 in]
            }
          }
          n238 = call-poly "Rack.vi"() -> ("error out"=w444:errorcluster, "Data Cluster"=w439:T1)  [unwired: 10 in]
          n239 = local write "InputData"(w439) -> ()
          n240 = control-ref of="Lickometer"() -> (w438:refnum<vi>)
          n241 = call-poly "Device.vi"("Device reference"=w438, "error in (no error)"=w444) -> ("Lick start?"=w441:bool)  [unwired: 7 in, 2 out]
          n242 = case shown="True" w441 {
            tunnel: w443 -> [w448 w449]
            tunnel: [w448 w453] -> w442
            frame False {
            }
            frame True {
              n243 = Unbundle By Name(w449) -> ("Licks"=w452:i32)
              n244 = Increment(x=w452) -> (x+1=w451:i32)
              n245 = Bundle By Name(cluster=w449, "Licks"=w451) -> (w453:T17)
              n246 = call "write-log.vi"("Write Text"=", 53, Internal, Lick, Speaker-2" ("text"), "Internal Cluster"=w449) -> ()  [unwired: 10 in]
            }
          }
          n247 = node-c288() -> ()  [unwired: 1 in, 1 out]
        }
        n248 = node-c288(w357) -> ()  [unwired: 1 out]
        n249 = node-c288(i64 2 ("Period")) -> (w361:T18)  [unwired: 3 in]
        n250 = Divide(x=w404, y=1000.0) -> (x/y=w433:dbl)
        n251 = Divide(x=w397, y=1000.0) -> (x/y=w398:dbl)
        n252 = timed-loop {
          tunnel: w433 -> [w496]
          tunnel: w406 -> [w512]
          shift-right: [w513] -> w376
          shift-left: w354 -> [w505]
          tunnel: w398 -> [w507]
          shift-right: [w510] -> w396
          shift-left: w425 -> [w511]
          shift-right: [w503] -> _
          shift-left: w374 -> [w504]
          tunnel: w373 -> [w502]
          timing: w361 -> [_]
          timing-out: [_] -> w360
          i -> [w509]
          stop <- w506 stop-if-true
          # "Min Lick Counter"
          # "Read licks"
          n253 = node-c288() -> ()  [unwired: 1 in, 1 out]
          n254 = control-ref of="Lickometer"() -> (w498:refnum<vi>)
          n255 = call-poly "Rack.vi"() -> ("error out"=w500:errorcluster, "Data Cluster"=→"InputData":T1)  [unwired: 10 in]
          n256 = call-poly "Device.vi"("Device reference"=w498, "error in (no error)"=w500) -> ("Lick start?"=w499:bool)  [unwired: 7 in, 2 out]
          n257 = case shown="False" w499 {
            tunnel: w504 -> [w517 w519]
            tunnel: [w517 w518] -> w503
            frame False {
            }
            frame True {
              n258 = Increment(x=w519) -> (x+1=w518:i32)
            }
          }
          n259 = call <vilib>:"High Resolution Relative Seconds.vi"() -> ("relative seconds"=w514:dbl)
          n260 = Greater Or Equal?(x=w503, y=w502) -> (x >= y?=w501:bool)
          n261 = Subtract(x=w514, y=w512) -> (x-y=w495:dbl)
          n262 = Subtract(x=w496, y=w495) -> (x-y=w494:dbl)
          n263 = local write "Time"(w494) -> ()
          n264 = Greater Or Equal?(x=w495, y=w496) -> (x >= y?=w506:bool)
          n265 = case shown="True" w506 {
            tunnel: w505 -> [_ w520]
            frame False {
            }
            frame True {
              # "Exit Log"
              n266 = stacked-sequence {
                tunnel: w520 -> [w521 w525]
                frame #0 {
                  n267 = call "write-log.vi"("Write Text"=", 94, Internal, End_Trial_Reception_Window, " ("text"), "Internal Cluster"=w521) -> ()  [unwired: 10 in]
                }
                frame #1 {
                  n268 = Unbundle By Name(w525) -> ("Next Trial"=w524:i32)
                  n269 = Equal To 0?(x=w524) -> (x = 0?=w523:bool)
                  n270 = case shown="True" w523 {
                    tunnel: w525 -> [_ _]
                    frame False {
                    }
                    frame True {
                    }
                  }
                }
              }
            }
          }
          n271 = Equal To 0?(x=w509) -> (x = 0?=w508:bool)
          n272 = case shown="True" w499 {
            tunnel: w505 -> [w532 w536]
            tunnel: [w532 w537] -> w513
            tunnel: w511 -> [w531 w535]
            tunnel: [w531 w534] -> w510
            tunnel: w501 -> [_ w533]
            frame False {
            }
            frame True {
              # "Write lick to log"
              n273 = case shown="True" w533 {
                tunnel: w536 -> [_ w545]
                tunnel: w535 -> [w541 w544]
                tunnel: [w541 w543] -> w534
                frame False {
                }
                frame True {
                  n274 = Unbundle By Name(w545) -> ("Next Trial"=w542:i32)
                  n275 = case shown="3" w542 {
                    tunnel: w544 -> [w547 w557 w567 w577]
                    tunnel: [w546 w556 w566 w576] -> w543
                    frame 0, Default {
                      # "Match"
                      n276 = Unbundle By Name(w547) -> ("Skip Receiving"=w548:bool)
                      n277 = case shown="False" w548 {
                        tunnel: w547 -> [w550 w555]
                        tunnel: [w549 w555] -> w546
                        frame False {
                          n278 = Bundle By Name(cluster=w550, "Trial Hit"=TRUE, "Trial Miss"=FALSE, "Trial FA"=FALSE ("Trial CR"), "Trial CR"=FALSE ("Trial FA")) -> (w549:T21)
                        }
                        frame True {
                        }
                      }
                    }
                    frame 1 {
                      # "Match"
                      n279 = Unbundle By Name(w557) -> ("Skip Receiving"=w558:bool)
                      n280 = case shown="False" w558 {
                        tunnel: w557 -> [w560 w565]
                        tunnel: [w559 w565] -> w556
                        frame False {
                          n281 = Bundle By Name(cluster=w560, "Trial Hit"=TRUE, "Trial Miss"=FALSE, "Trial FA"=FALSE ("Trial CR"), "Trial CR"=FALSE ("Trial FA")) -> (w559:T21)
                        }
                        frame True {
                        }
                      }
                    }
                    frame 2 {
                      # "Non-match"
                      n282 = Unbundle By Name(w567) -> ("Skip Receiving"=w568:bool)
                      n283 = case shown="False" w568 {
                        tunnel: w567 -> [w570 w575]
                        tunnel: [w569 w575] -> w566
                        frame False {
                          n284 = Bundle By Name(cluster=w570, "Trial Hit"=FALSE, "Trial Miss"=FALSE, "Trial FA"=TRUE ("Trial CR"), "Trial CR"=FALSE ("Trial FA")) -> (w569:T21)
                        }
                        frame True {
                        }
                      }
                    }
                    frame 3 {
                      # "Non-match"
                      n285 = Unbundle By Name(w577) -> ("Skip Receiving"=w578:bool)
                      n286 = case shown="False" w578 {
                        tunnel: w577 -> [w580 w585]
                        tunnel: [w579 w585] -> w576
                        frame False {
                          n287 = Bundle By Name(cluster=w580, "Trial Hit"=FALSE, "Trial Miss"=FALSE, "Trial FA"=TRUE ("Trial CR"), "Trial CR"=FALSE ("Trial FA")) -> (w579:T21)
                        }
                        frame True {
                        }
                      }
                    }
                  }
                }
              }
              n288 = Unbundle By Name(w536) -> ("Licks"=w539:i32)
              n289 = Increment(x=w539) -> (x+1=w538:i32)
              n290 = Bundle By Name(cluster=w536, "Licks"=w538) -> (w537:T17)
              n291 = call "write-log.vi"("Write Text"=", 52, Internal, Lick, Trial_Reception_Window" ("text"), "Internal Cluster"=w536) -> ()  [unwired: 10 in]
            }
          }
          n292 = case shown="True" w508 {
            tunnel: w505 -> [_ w530]
            tunnel: w507 -> [_ w526]
            frame False {
            }
            frame True {
              n293 = Number To Fractional String(number=w526) -> (F-format string=w527:string)  [unwired: 3 in]
              n294 = Concatenate Strings(", 92, Internal, Start_Trial_Reception_Window, " ("text"), w527) -> (w529:string)
              n295 = call "write-log.vi"("Write Text"=w529, "Internal Cluster"=w530) -> ()  [unwired: 10 in]
            }
          }
          n296 = node-c288() -> ()  [unwired: 1 in, 1 out]
        }
        n297 = Unbundle By Name(w396) -> ("Trial Hit"=w353:bool, "Trial Miss"=w409:bool, "Trial FA"=w408:bool, "Trial CR"=w407:bool)
        n298 = case shown="True" TRUE {
          tunnel: w376 -> [w718 w726]
          tunnel: [w718 w725] -> w368
          tunnel: w370 -> [_ w721]
          frame False {
          }
          frame True {
            n299 = Unbundle By Name(w726) -> ("Reward Dispensed"=w728:dbl)
            n300 = Add(x=w728, y=w721) -> (x+y=w727:dbl)
            n301 = Bundle By Name(cluster=w726, "Reward Dispensed"=w727) -> (w725:T17)
            n302 = Number To Fractional String(number=w721) -> (F-format string=w722:string)  [unwired: 3 in]
            n303 = Concatenate Strings(", 100, External, Dispense_Reward," ("text"), w722) -> (w724:string)
            n304 = call "write-log.vi"("Write Text"=w724, "Internal Cluster"=w726) -> ()  [unwired: 10 in]
            n305 = control-ref of="Valve"() -> (w720:refnum<vi>)
            n306 = call-poly "Device.vi"("Device reference"=w720, "Duration"=0) -> ()  [unwired: 8 in, 2 out]
          }
        }
        n307 = Or(x=w409, y=w408) -> (x .or. y?=w402:bool)
        n308 = Unbundle By Name(w368) -> ("Hits"=w424:i32, "Miss"=w423:i32, "False Alarm"=w418:i32, "Correct Rejection"=w422:i32)
        n309 = Boolean To (0,1)(Boolean=w353) -> (0, 1=w419:i16)
        n310 = Boolean To (0,1)(Boolean=w409) -> (0, 1=w420:i16)
        n311 = Boolean To (0,1)(Boolean=w408) -> (0, 1=w417:i16)
        n312 = Boolean To (0,1)(Boolean=w407) -> (0, 1=w421:i16)
        n313 = Add(x=w419, y=w424) -> (x+y=w414:i32)
        n314 = Add(x=w417, y=w418) -> (x+y=w416:i32)
        n315 = Add(x=w420, y=w423) -> (x+y=w415:i32)
        n316 = Add(x=w421, y=w422) -> (x+y=w413:i32)
        n317 = Compound Arithmetic op=ADD(w414, w413) -> (w412:i32)
        n318 = Compound Arithmetic op=ADD(w414, w415, w416, w413) -> (w411:i32)
        n319 = Divide(x=w412, y=w411) -> (x/y=w410:dbl)
        n320 = Unbundle By Name(w396) -> ("Trial Hit"=w395:bool, "Trial Miss"=w386:bool, "Trial FA"=w385:bool, "Trial CR"=w384:bool)
        n321 = Bundle By Name(cluster=w368, "Hits"=w414, "Miss"=w415, "False Alarm"=w416, "Correct Rejection"=w413, "Accuracy"=w410, "Punish ITI"=w402) -> (w378:T17)
        n322 = Select(t=", 62, Internal, Trial_FA," ("text"), s=w385, f="") -> (s? t:f=w381:string)
        n323 = Select(t=", 60, Internal, Trial_Hit," ("text"), s=w395, f="") -> (s? t:f=w383:string)
        n324 = Select(t=", 61, Internal, Trial_Miss," ("text"), s=w386, f="") -> (s? t:f=w382:string)
        n325 = Select(t=", 63, Internal, Trial_CR," ("text"), s=w384, f="") -> (s? t:f=w380:string)
        n326 = Concatenate Strings(w383, w382, w381, w380) -> (w379:string)
        n327 = stacked-sequence {
          tunnel: w379 -> [w698 _]
          tunnel: w378 -> [w697 w701]
          tunnel: [_ w700] -> w369
          tunnel: [_ w699] -> _
          tunnel: w352 -> [_ w699]
          frame #0 {
            # "Trial_"
            n328 = call "write-log.vi"("Write Text"=w698, "Internal Cluster"=w697) -> ()  [unwired: 10 in]
          }
          frame #1 {
            n329 = case shown="3" w699 {
              tunnel: w701 -> [w702 w704 w706 w708]
              tunnel: [w702 w704 w706 w708] -> w700
              frame 0, Default {
                n330 = call "write-log.vi"("Write Text"=", 97, Internal, End_Match_Trial, " ("text"), "Internal Cluster"=w702) -> ()  [unwired: 10 in]
              }
              frame 1 {
                n331 = call "write-log.vi"("Write Text"=", 97, Internal, End_Match_Trial, " ("text"), "Internal Cluster"=w704) -> ()  [unwired: 10 in]
              }
              frame 2 {
                n332 = call "write-log.vi"("Write Text"=", 98, Internal, End_Nonmatch_Trial, " ("text"), "Internal Cluster"=w706) -> ()  [unwired: 10 in]
              }
              frame 3 {
                n333 = call "write-log.vi"("Write Text"=", 98, Internal, End_Nonmatch_Trial, " ("text"), "Internal Cluster"=w708) -> ()  [unwired: 10 in]
              }
            }
          }
        }
        n334 = node-c288(w360) -> ()  [unwired: 1 out]
        n335 = Select(t="Punish ITI", s=w402, f="ITI") -> (s? t:f=w403:string)
      }
      frame "Stop" {
        n336 = call "write-log.vi"("Write Text"=", 110, External, End_Session_Trials_Finished, " ("text"), "Internal Cluster"=w746) -> ()  [unwired: 10 in]
      }
    }
    "Current State" <- w268
    n337 = Unbundle By Name(w246) -> ("relative seconds"=w273:dbl)
    n338 = Unbundle By Name(w267) -> ("Max Time (s)"=w272:dbl)
    n339 = call <vilib>:"High Resolution Relative Seconds.vi"() -> ("relative seconds"=w274:dbl)
    n340 = Subtract(x=w274, y=w273) -> (x-y=w270:dbl)
    "Time Elapsed" <- w270
    n341 = Greater Or Equal?(x=w270, y=w272) -> (x >= y?=w244:bool)
    n342 = Or(x="stop", y=w244) -> (x .or. y?=w242:bool)
    n343 = Or(x=w271, y=w242) -> (x .or. y?=w247:bool)
    n344 = case shown="True" w242 {
      tunnel: w246 -> [_ w276]
      frame False {
      }
      frame True {
        n345 = call "write-log.vi"("Write Text"=", 111, External, End_Session_Time_Reached, " ("text"), "Internal Cluster"=w276) -> ()  [unwired: 10 in]
      }
    }
    n346 = Unbundle By Name(w266) -> ("Accuracy"=→"Acc":dbl, "Hits"=w253:i32, "Miss"=w254:i32, "False Alarm"=w255:i32, "Correct Rejection"=w256:i32, "Current Trial Index"=w249:i32, "Licks"=w257:i32, "Reward Dispensed"=w258:dbl)
    n347 = Number To Decimal String(number=w257) -> (decimal integer string=→"Licks":string)  [unwired: 1 in]
    n348 = Number To Fractional String(number=w258) -> (F-format string=→"Reward Dispensed (uL)":string)  [unwired: 3 in]
    n349 = Decrement(x=w249) -> (x-1=w250:i32)
    n350 = Number To Decimal String(number=w253) -> (decimal integer string=→"Hits":string)  [unwired: 1 in]
    n351 = Number To Decimal String(number=w254) -> (decimal integer string=→"Miss":string)  [unwired: 1 in]
    n352 = Number To Decimal String(number=w255) -> (decimal integer string=→"FA":string)  [unwired: 1 in]
    n353 = Number To Decimal String(number=w256) -> (decimal integer string=→"CR":string)  [unwired: 1 in]
    n354 = Number To Decimal String(number=w250) -> (decimal integer string=→"Trials":string)  [unwired: 1 in]
  }
  n355 = Concatenate Strings(w110, w109, w108, w107, w106, w105, w48, w42, w30, w29) -> (w102:string)
  n356 = Write to Text File(file (use dialog)=w104, text=w102) -> (refnum out=w103:refnum<file>)  [unwired: 2 in, 2 out]
  n357 = Concatenate Strings("Match_Delay_Lick,NA\nMatch_Reception_Lick,Hit\nMatch_No_Lick,Miss\nNonmatch_Delay_Lick,NA\nNonmatch_Reception_Lick,False_Alarm\nNonmatch_No_Lick,Correct_Reject", "\r\n") -> (w138:string)
  n358 = Write to Text File(file (use dialog)=w103, text=w138) -> (refnum out=w139:refnum<file>)  [unwired: 2 in, 2 out]
  n359 = Concatenate Strings("Trial_Sequence," ("string"), w140, "\r\n") -> (w172:string)
  n360 = Write to Text File(file (use dialog)=w139, text=w172) -> (refnum out=w173:refnum<file>)  [unwired: 2 in, 2 out]
  n361 = Write to Text File(file (use dialog)=w173, text="\r\n") -> (refnum out=w179:refnum<file>)  [unwired: 2 in, 2 out]
  n362 = Concatenate Strings("----------" ("string"), "\r\n") -> (w178:string)
  n363 = Write to Text File(file (use dialog)=w179, text=w178) -> (refnum out=w145:refnum<file>)  [unwired: 2 in, 2 out]
  n364 = Concatenate Strings("Time, ID, Type, Name, Value" ("string"), "\r\n") -> (w143:string)
  n365 = Write to Text File(file (use dialog)=w145, text=w143) -> (refnum out=w144:refnum<file>)  [unwired: 2 in, 2 out]
  n366 = Close File(refnum=w144) -> ()  [unwired: 1 in, 2 out]
  n367 = Unbundle By Name(w60) -> ("appended path"=w55:path, "Accuracy"=w95:dbl, "Hits"=w94:i32, "Miss"=w93:i32, "False Alarm"=w92:i32, "Correct Rejection"=w91:i32, "Licks"=w90:i32, "Reward Dispensed"=w89:dbl)
  n368 = control-ref of="Lickometer"() -> (w22:refnum<vi>)
  n369 = call-poly "Rack.vi"("OutputRequest channel"=w20) -> ("error out"=w24:errorcluster)  [unwired: 10 in]
  n370 = call-poly "Device.vi"("Device reference"=w22, "error in (no error)"=w24) -> ()  [unwired: 9 in, 1 out]
  n371 = Number To Decimal String(number=w90) -> (decimal integer string=w77:string)  [unwired: 1 in]
  n372 = Number To Decimal String(number=w89) -> (decimal integer string=w75:string)  [unwired: 1 in]
  n373 = Number To Decimal String(number=w91) -> (decimal integer string=w79:string)  [unwired: 1 in]
  n374 = Number To Decimal String(number=w93) -> (decimal integer string=w83:string)  [unwired: 1 in]
  n375 = Number To Decimal String(number=w92) -> (decimal integer string=w81:string)  [unwired: 1 in]
  n376 = Number To Decimal String(number=w94) -> (decimal integer string=w85:string)  [unwired: 1 in]
  n377 = Number To Fractional String(number=w95) -> (F-format string=w88:string)  [unwired: 3 in]
  n378 = Concatenate Strings("-1, 120, External, End_Session_Accuracy, " ("text"), w88, "\r\n") -> (w67:string)
  n379 = Concatenate Strings("-1, 125, External, End_Session_Number_Licks, " ("text"), w77, "\r\n") -> (w62:string)
  n380 = Concatenate Strings("-1, 126, External, End_Session_Reward_Dispensed_ml, " ("text"), w75, "\r\n") -> (w61:string)
  n381 = Concatenate Strings("-1, 124, External, End_Session_Number_CR, " ("text"), w79, "\r\n") -> (w63:string)
  n382 = Concatenate Strings("-1, 121, External, End_Session_Number_Hits, " ("text"), w85, "\r\n") -> (w66:string)
  n383 = Concatenate Strings("-1, 122, External, End_Session_Number_Miss, " ("text"), w83, "\r\n") -> (w65:string)
  n384 = Concatenate Strings("-1, 123, External, End_Session_Number_FA, " ("text"), w81, "\r\n") -> (w64:string)
  n385 = Concatenate Strings(w67, w66, w65, w64, w63, w62, w61) -> (w54:string)
  n386 = Open/Create/Replace File(file path (use dialog)=w55) -> (refnum out=w57:refnum<file>)  [unwired: 5 in, 2 out]
  n387 = Set File Position(refnum=w57, from (0:start)=enum16{"start", "end", "current"}."end") -> (refnum out=w59:refnum<file>)  [unwired: 2 in, 1 out]
  n388 = Write to Text File(file (use dialog)=w59, text=w54) -> (refnum out=w56:refnum<file>)  [unwired: 2 in, 2 out]
  n389 = Close File(refnum=w56) -> ()  [unwired: 1 in, 2 out]
